vi "MIIPS Mask Apply v2.vi"(4 "SLM COM Port":refnum<visa-resource-name>="COM9", 8 "Master Mask Calibration":path=path "C:/Alexander/LabView programs/SLM/Calibration Data/230712 master mask.txt", 9 "Slave Mask Calibration":path=path "C:/Alexander/LabView programs/SLM/Calibration Data/230712 slave mask.txt", 10 "Phase":dbl[](array[numeric]), 11 "Wavelength":dbl[](array[numeric])) -> (1 "Applied":bool, 2 "Interpolated phase":dbl[](array[numeric]) format="%_6g", 3 "Sampled wavelengths":dbl[](array[numeric]) format="%_6g")   [LabVIEW 2022 SP3]
uses:
  <vilib>/Utility/file.llb/Read Delimited Spreadsheet (DBL).vi
  Global 1.vi
  <vilib>/gmath/NI_Gmath.lvlib
panel:
  out "Slave":cluster{dbl, i32, dbl[]}(graph)
  out "Master":cluster{dbl, i32, dbl[]}(graph)
  in  "Boolean":bool=TRUE
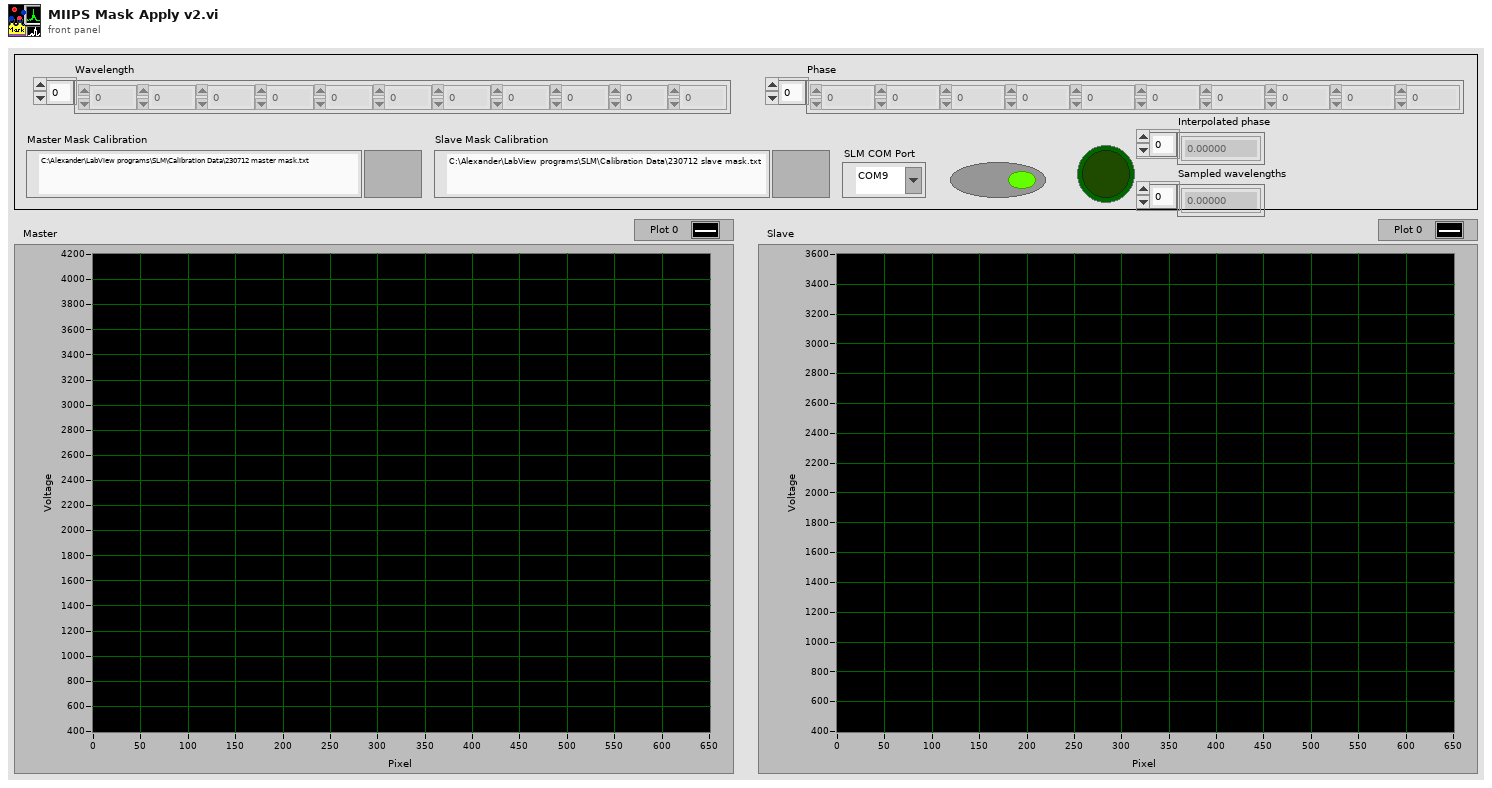
[diagram p1: front panel]
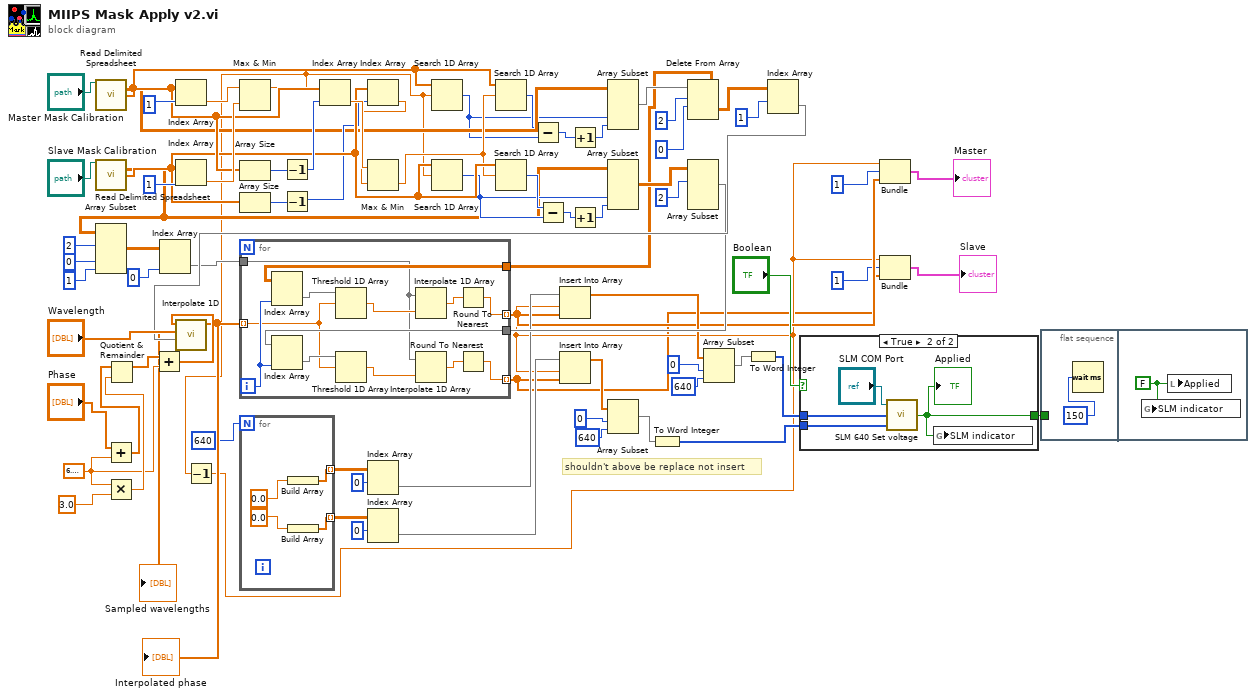
[diagram p0: block diagram]
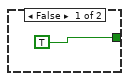
[diagram p2: hidden frame]
diagram:
  w37 = 6.283185307179586
  # "shouldn't above be replace not insert"
  n1 = call-poly <vilib>:"Read Delimited Spreadsheet.vi"("file path (dialog if empty)"="Master Mask Calibration") -> ("all rows"=w63:dbl[][], "first row"=w67:dbl[])  [unwired: 9 in, 4 out]
  n2 = call-poly <vilib>:"Read Delimited Spreadsheet.vi"("file path (dialog if empty)"="Slave Mask Calibration") -> ("all rows"=w54:dbl[][], "first row"=w66:dbl[])  [unwired: 9 in, 4 out]
  n3 = Array Subset(array=w54, index (row)=2 ("index"), index (col)=0 ("index"), length (col)=1 ("length")) -> (w50:dbl[][])  [unwired: 1 in]
  n4 = Add(x="Phase", y=w37) -> (x+y=w41:dbl[])
  n5 = Multiply(x=w37, y=3.0) -> (x*y=w39:dbl)
  n6 = Quotient & Remainder(x=w41, y=w39) -> (x-y*floor(x/y)=w38:dbl[])  [unwired: 1 out]
  n7 = Add(x=w38, y=w37) -> (x+y=w36:dbl[])
  n8 = Index Array(array=w50, index (col)=0 ("index (row)")) -> (element=w30:dbl[])  [unwired: 1 in]
  n9 = Index Array(array=w67, index=1 ("index (row)")) -> (element=w75:dbl)
  n10 = Index Array(array=w66, index=1) -> (element=w74:dbl)
  n11 = Max & Min(x=w75, y=w74) -> (max(x,y)=w24:dbl)  [unwired: 1 out]
  n12 = Decrement(x=w24) -> (x-1=w5:dbl)
  n13 = Array Size(array=w67) -> (size(s)=w72:i32)
  n14 = Array Size(array=w66) -> (size(s)=w71:i32)
  n15 = for {
    N: 640 -> [_]
    tunnel: [w80] -> w26 mode=indexing
    tunnel: [w79] -> w25 mode=indexing
    n16 = Build Array(0.0 ("element")) -> (w80:dbl[])
    n17 = Build Array(0.0 ("element")) -> (w79:dbl[])
  }
  n18 = Decrement(x=w72) -> (x-1=w70:i32)
  n19 = Decrement(x=w71) -> (x-1=w65:i32)
  n20 = Index Array(array=w67, index=w70) -> (element=w69:dbl)
  n21 = Index Array(array=w66, index=w65) -> (element=w68:dbl)
  n22 = Max & Min(x=w69, y=w68) -> (min(x,y)=w64:dbl)  [unwired: 1 out]
  n23 = Index Array(array=w26, index (col)=0 ("index (row)")) -> (element=w21:dbl[])  [unwired: 1 in]
  n24 = Index Array(array=w25, index (col)=0 ("index (row)")) -> (element=w22:dbl[])  [unwired: 1 in]
  n25 = Search 1D Array(1D array=w67, element=w24) -> (index of element=w61:i32)  [unwired: 1 in]
  n26 = Search 1D Array(1D array=w66, element=w24) -> (index of element=w59:i32)  [unwired: 1 in]
  n27 = Search 1D Array(1D array=w67, element=w64) -> (index of element=w62:i32)  [unwired: 1 in]
  n28 = Search 1D Array(1D array=w66, element=w64) -> (index of element=w60:i32)  [unwired: 1 in]
  n29 = Subtract(x=w62, y=w61) -> (x-y=w58:i32)
  n30 = Subtract(x=w60, y=w59) -> (x-y=w56:i32)
  n31 = Increment(x=w58) -> (x+1=w57:i32)
  n32 = Increment(x=w56) -> (x+1=w55:i32)
  n33 = Array Subset(array=w63, index (col)=w61, length (col)=w57) -> (w49:dbl[][])  [unwired: 2 in]
  n34 = Array Subset(array=w54, index (col)=w59, length (col)=w55) -> (w46:dbl[][])  [unwired: 2 in]
  n35 = Delete From Array(array=w49, length=2, index (row)=0) -> (deleted portion=w44:dbl[][], array with subset deleted=w31:dbl[][])  [unwired: 1 in]
  n36 = Array Subset(array=w46, index (row)=2 ("index")) -> (w32:dbl[][])  [unwired: 3 in]
  n37 = Index Array(array=w44, index (row)=1) -> (element=w34:dbl[])  [unwired: 1 in]
  n38 = call <vilib>:"Interpolate 1D.vi"("xi"=w34, "X"="Wavelength", "Y"=w36) -> ("xi used"=→"Sampled wavelengths":dbl[], "yi"=w33:dbl[])  [unwired: 6 in, 1 out]
  "Interpolated phase" <- w33
  n39 = for {
    tunnel: w33 -> [w90] mode=indexing
    tunnel: w32 -> [w95]
    tunnel: w31 -> [w94]
    tunnel: w30 -> [w87]
    tunnel: [w84] -> w9 mode=indexing
    tunnel: [w83] -> w4 mode=indexing
    i -> [w93]
    n40 = Index Array(array=w94, index (col)=w93) -> (element=w92:dbl[])  [unwired: 1 in]
    n41 = Index Array(array=w95, index (col)=w93) -> (element=w91:dbl[])  [unwired: 1 in]
    n42 = Threshold 1D Array(2:w90, 3:w92) -> (0:w89:dbl)  [unwired: 1 in]
    n43 = Threshold 1D Array(2:w90, 3:w91) -> (0:w88:dbl)  [unwired: 1 in]
    n44 = Interpolate 1D Array(1:w89, 2:w87) -> (0:w86:dbl)
    n45 = Interpolate 1D Array(1:w88, 2:w87) -> (0:w85:dbl)
    n46 = Round To Nearest(number=w86) -> (nearest integer value=w84:dbl)
    n47 = Round To Nearest(number=w85) -> (nearest integer value=w83:dbl)
  }
  n48 = Insert Into Array(array=w21, index=w5, new element=w9) -> (w20:dbl[])
  n49 = Insert Into Array(array=w22, index=w5, new element=w4) -> (w16:dbl[])
  n50 = Array Subset(array=w16, index=0, length=640) -> (w14:dbl[])
  n51 = To Word Integer(number=w14) -> (16bit integer=w12:i16[])
  n52 = Array Subset(array=w20, index=0, length=640) -> (w15:dbl[])
  n53 = To Word Integer(number=w15) -> (16bit integer=w13:i16[])
  n54 = case shown="True" "Boolean" {
    tunnel: w13 -> [_ w99]
    tunnel: w12 -> [_ w98]
    tunnel: [TRUE w97] -> w3
    frame False {
    }
    frame True {
      n55 = call "SLM 640 Set voltage.vi"("Slave"=w98, "Master"=w99, "VISA Resource Name"="SLM COM Port") -> ("Normal?"=w97:bool)  [unwired: 2 out]
      "Applied" <- w97
      n56 = global write "Global 1.vi" "SLM indicator"(w97) -> ()
    }
  }
  n57 = Bundle(w5, 1, w9) -> (→"Master":cluster{dbl, i32, dbl[]})  [unwired: 1 in]
  n58 = Bundle(w5, 1, w4) -> (→"Slave":cluster{dbl, i32, dbl[]})  [unwired: 1 in]
  n59 = flat-sequence {
    tunnel: w3 -> [_]
    frame #0 {
      n60 = Wait (ms)(milliseconds to wait=u32 150) -> ()  [unwired: 1 out]
    }
    frame #1 {
      w102 = FALSE ("Applied")
      n61 = global write "Global 1.vi" "SLM indicator"(w102) -> ()
      n62 = local write "Applied"(w102) -> ()
    }
  }
